vi "Get .Net Container.vi"(11 "SourceGrid in":refnum<class "SourceGrid.lvclass">) -> (2 ".NET Container":refnum<k24>, 3 "SourceGrid out":refnum<class "SourceGrid.lvclass">)   [LabVIEW 2024, in "SourceGrid.lvlib" / "SourceGrid.lvclass"]
uses:
  SourceGrid.lvclass
  SourceGrid.lvclass/SourceGrid.ctl
  D:/git/Sourcegrid-LabVIEW/dll/SourceGrid.dll
  dll/SourceGrid.dll
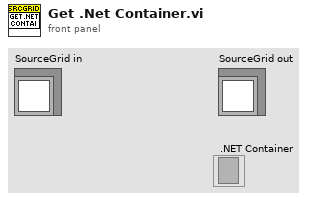
[diagram p1: front panel]
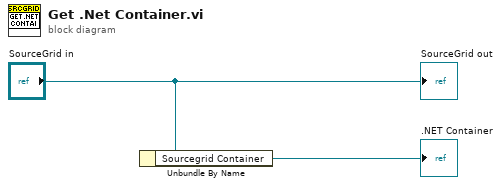
[diagram p0: block diagram]
diagram:
  n1 = Unbundle By Name("SourceGrid in") -> ("Sourcegrid Container"=→".NET Container":refnum<k24>)
  "SourceGrid out" <- "SourceGrid in"
